vi "ReadString.vi"(8 "Uart Input":cluster{u64}={185291944} {"?" format="%x"}, 11 "Error Input":errorcluster) -> (0 "Uart Output":cluster{u64}={185291944} {"?" format="%x"}, 1 "String Length":u32=10, 2 "String Data":string="ECC-Lab.\r\n", 3 "Error Output":errorcluster)   [LabVIEW 2019]
doc: "<B>Read</B> internal bytes buffer of the serial port. The internal bytes buffer will be cleared automatically."
uses:
  dll/LabViewUart.dll
panel:
  # "Read String Data"
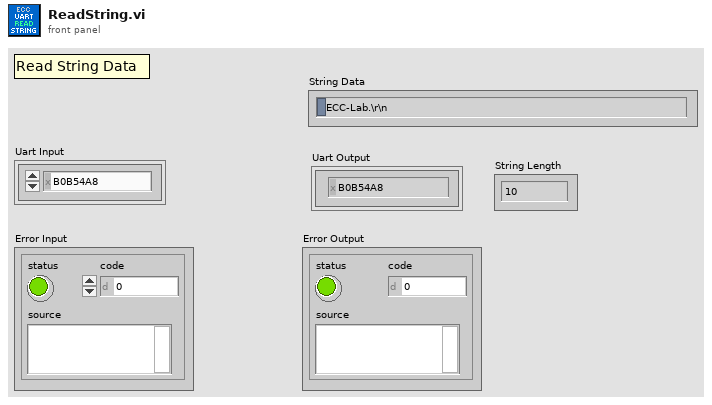
[diagram p1: front panel]
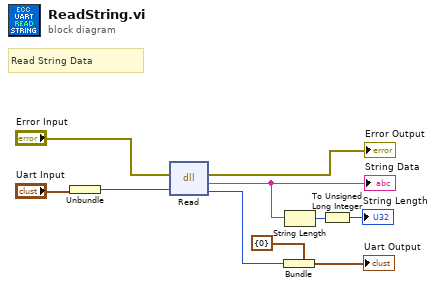
[diagram p0: block diagram]
diagram:
  # "Read String Data"
  n1 = Unbundle("Uart Input") -> (w7:u64)
  n2 = dll-call lib="D:/Google Drive/INC-2020/INC352/INC352-2020/LabVIEW/examples/uart-cmdex/SubVI/dll/LabViewUart.dll" fn="Read"(error in="Error Input", "Uart Handle"=w7) -> (error out=→"Error Output":errorcluster, "String Data"=w3:string, "Uart Handle"=w4:u64)  [unwired: 2 in, 1 out]
  "String Data" <- w3
  n3 = Bundle(cluster=cluster{u64} {0}, w4) -> (→"Uart Output":cluster{u64})
  n4 = String Length(string=w3) -> (length=w2:i32)
  n5 = To Unsigned Long Integer(number=w2) -> (unsigned 32bit integer=→"String Length":u32)
